vi "TTTR.vi"(4 "error in (no error)":errorcluster, 5 "file refnum":refnum<file>, 6 "Array":u8[](array[numeric]), 7 "DeviceIndex":i32) -> (0 "count":i32, 1 "error out":errorcluster, 2 "FiFoOverrun":bool, 3 "OK":bool)   [LabVIEW 2011]
uses:
  MT Scan/SubVIs/hhlib.dll
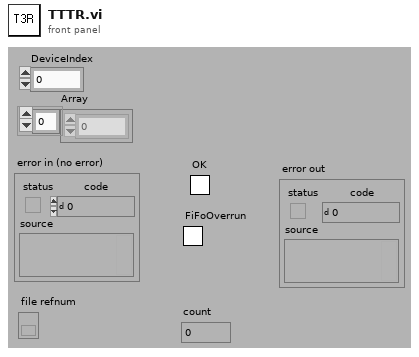
[diagram p1: front panel]
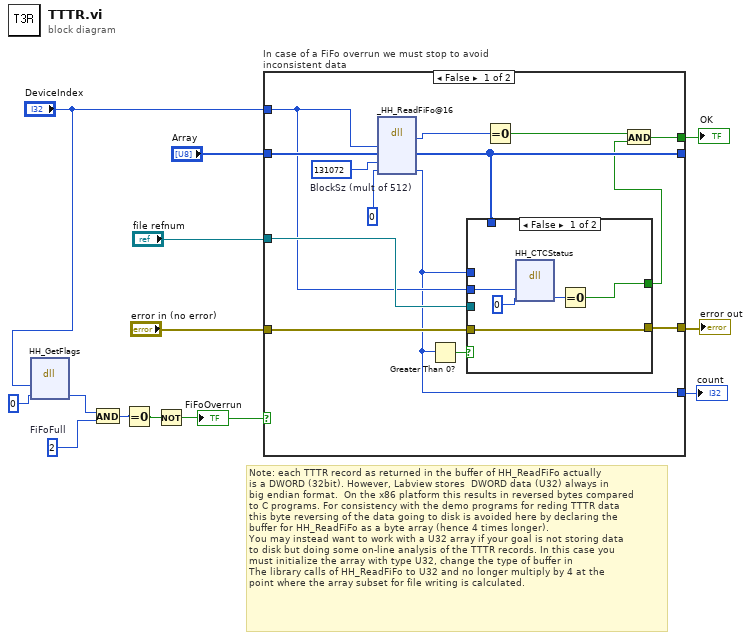
[diagram p0: block diagram]
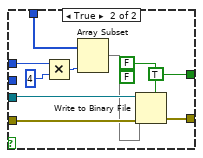
[diagram p2: hidden frame]
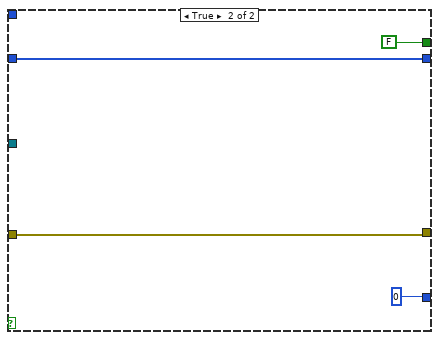
[diagram p3: hidden frame]
diagram:
  w8 = 2  # FiFoFull
  # "Note: each TTTR record as returned in the buffer of HH_ReadFiFo actually \nis a DWORD (32bit). However, Labview stores  DWORD data (U32) always in \nbig endian format.  On the x86 platform this results in reversed bytes compared \nto C programs. For consistency with the demo programs for reding TTTR data \nthis byte reversing of the data going to disk is avoided here by declaring the \nbuffer for HH_ReadFiFo as a byte array (hence 4 times longer).\nYou may instead want to work with a U32 array if your goal is not storing data \nto disk but doing some on-line analysis of the TTTR records. In this case you \nmust initialize the array with type U32, change the type of buffer in\nThe library calls of HH_ReadFiFo to U32 and no longer multiply by 4 at the \npoint where the array subset for file writing is calculated."
  n1 = dll-call lib="C:/Users/Core-FCS/Desktop/AbelFCS/MT Scan/SubVIs/hhlib.dll" fn="HH_GetFlags"("devidx"="DeviceIndex", "flags"=0) -> ("flags"=w1:i32)  [unwired: 5 in, 2 out]
  n2 = And(x=w1, y=w8) -> (x .and. y?=w7:i32)
  n3 = Equal To 0?(x=w7) -> (x = 0?=w6:bool)
  n4 = Not ("CTCDone")(x=w6) -> (.not. x?=w5:bool)
  "FiFoOverrun" <- w5
  n5 = case "In case of a FiFo overrun we must stop to avoid inconsistent data" shown="False" w5 {
    tunnel: "Array" -> [w22 w45]
    tunnel: [w16 0] -> w13
    tunnel: [w21 w45] -> _
    tunnel: [w27 w44] -> w12
    tunnel: "error in (no error)" -> [w25 w44]
    tunnel: [w23 FALSE] -> w10
    tunnel: "file refnum" -> [w26 _]
    tunnel: "DeviceIndex" -> [w19 _]
    frame False {
      w20 = 131072  # BlockSz (mult of 512)
      n6 = dll-call lib="C:/Users/Core-FCS/Desktop/AbelFCS/MT Scan/SubVIs/hhlib.dll" fn="_HH_ReadFiFo@16" label="HH_ReadFiFo"("devidx"=w19, "buffer"=w22, "blocksize"=w20, "nactual"=0) -> (w17:i32, "buffer"=w21:u8[], "nactual"=w16:i32)  [unwired: 5 in, 2 out]
      n7 = Greater Than 0?(x=w16) -> (x > 0?=w24:bool)
      n8 = case shown="False" w24 {
        tunnel: [w32 w42] -> w27
        tunnel: w26 -> [_ w41]
        tunnel: w25 -> [w32 w40]
        tunnel: [w31 TRUE] -> w14
        tunnel: w21 -> [_ w38]
        tunnel: w16 -> [_ w35]
        tunnel: w19 -> [w30 _]
        frame False {
          n9 = dll-call lib="C:/Users/Core-FCS/Desktop/AbelFCS/MT Scan/SubVIs/hhlib.dll" fn="HH_CTCStatus"("devidx"=w30, "status"=0) -> ("status"=w28:i32)  [unwired: 5 in, 2 out]
          n10 = Equal To 0?(x=w28) -> (x = 0?=w31:bool)
        }
        frame True {
          (unwired) FALSE ("prepend array or string size? (T)")
          n11 = Multiply(x=w35, y=4) -> (x*y=w36:i32)
          n12 = Array Subset(array=w38, length=w36) -> (w37:u8[])  [unwired: 1 in]
          n13 = Write to Binary File(file (use dialog)=w41, data=w37, error in=w40, 5:FALSE ("Array- oder String-Größe voranstellen? (T)")) -> (error out=w42:errorcluster)  [unwired: 2 in, 2 out]
        }
      }
      n14 = Equal To 0?(x=w17) -> (x = 0?=w15:bool)
      n15 = And(x=w15, y=w14) -> (x .and. y?=w23:bool)
    }
    frame True {
    }
  }
  "OK" <- w10
  "count" <- w13
  "error out" <- w12
